vi "delete one digital.vi"(8 "error in (no error)":errorcluster) -> (0 "error out":errorcluster)   [LabVIEW 2020, in "Settings.lvlib"]
uses:
  Settings.lvlib
  <vilib>/drjdpowell/SQLite Library/SQL Connection/Open (path).vi
  <vilib>/drjdpowell/SQLite Library/SQL Connection/Open (string).vi
  <vilib>/AdvancedString/Path To Command Line String.vi
  <vilib>/drjdpowell/SQLite Library/SQL Connection/Execute SQL (No results).vi
  <vilib>/drjdpowell/SQLite Library/SQL Connection/Connection.lvclass
  <vilib>/drjdpowell/SQLite Library/SQLite.lvlib
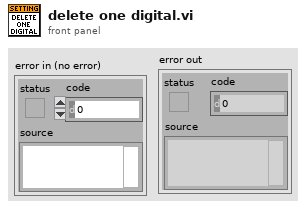
[diagram p1: front panel]
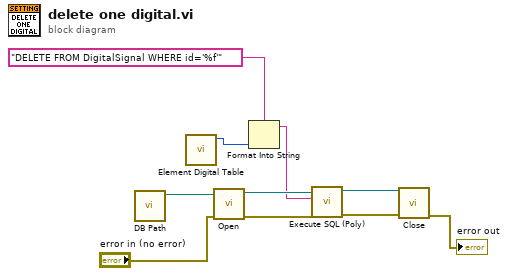
[diagram p0: block diagram]
diagram:
  n1 = call "DB Path.vi"() -> ("DB path"=w2:path)  [unwired: 11 in]
  n2 = call "Element Digital Table.vi"() -> ("element"=w1:i64)  [unwired: 10 in, 1 out]
  n3 = call-poly <vilib>:"Open.vi"("error in (no error)"="error in (no error)", "db file"=w2) -> ("error out"=w10:errorcluster, "SQLite Connection"=w8:refnum<class "Connection.lvclass">)  [unwired: 8 in]
  n4 = Format Into String(format string="DELETE FROM DigitalSignal WHERE id='%f'" ("SQL"), w1) -> (resulting string=w4:string)  [unwired: 2 in, 1 out]
  n5 = call-poly <vilib>:"Execute SQL (Poly).vi"("error in (no error)"=w10, "SQL"=w4, "SQLite Connection in"=w8) -> ("error out"=w9:errorcluster, "SQLite Connection"=w7:refnum<class "Connection.lvclass">)  [unwired: 7 in]
  n6 = call-dynamic "Close.vi"("error in (no error)"=w9, "SQLite Connection in"=w7) -> ("error out"=→"error out":errorcluster)  [unwired: 9 in]
